vi "Set_CC_Get_Voltage.vi"(7 "Stop Maker 2":dbl=3.0 format="%#_13g", 8 "error in (no error)":errorcluster, 9 "Limit (1.0 A)":dbl=-0.2 format="%.10f", 10 "Channel Name (1)":string, 11 "VISA Refnum in":refnum<visa-resource-name>) -> (0 "error out":errorcluster {"code" format="%.0x"}, 1 "Current Measurement":dbl format="%.10f", 2 "Voltage Measurement":dbl format="%.3f", 3 "VISA Refnum out":refnum<visa-resource-name>)   [LabVIEW 2015]
uses:
  <instrlib>/Agilent N6700 Series/Agilent N6700 Series.lvlib
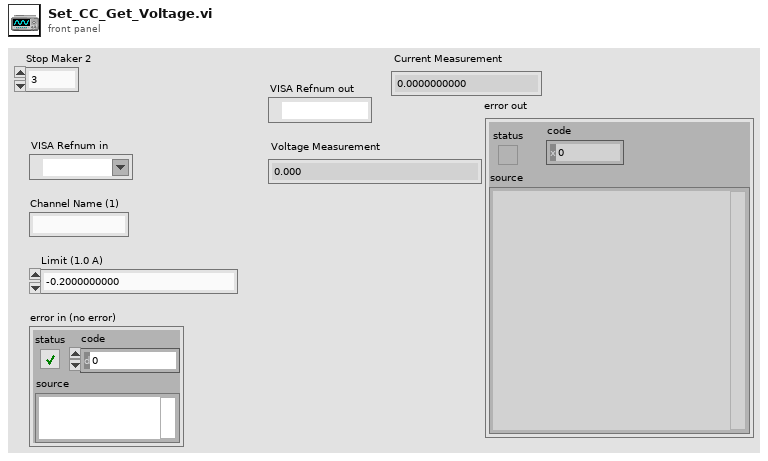
[diagram p1: front panel]
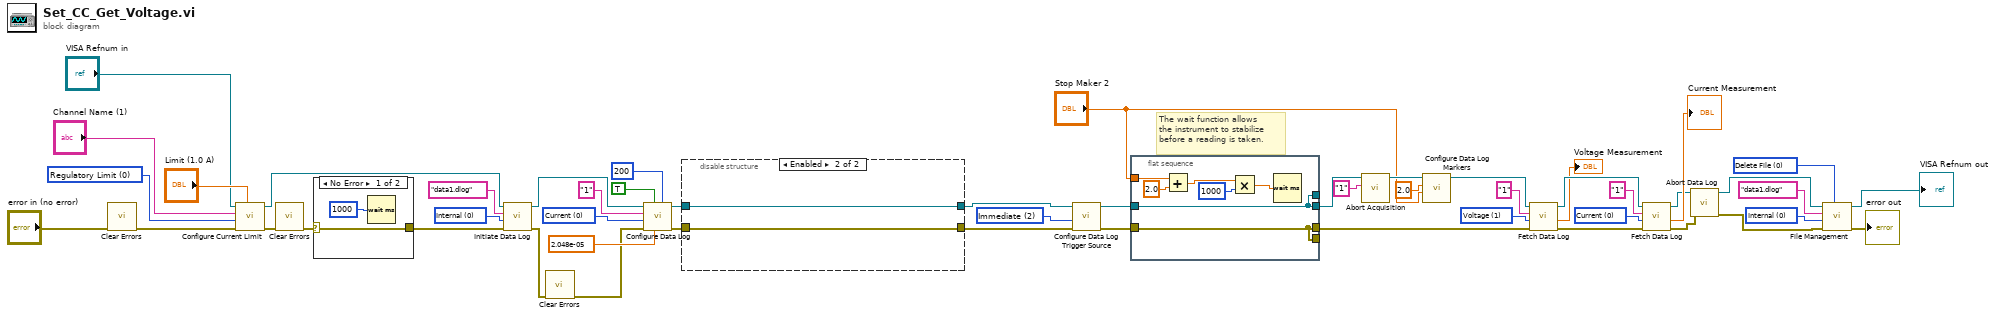
[diagram p0: block diagram]
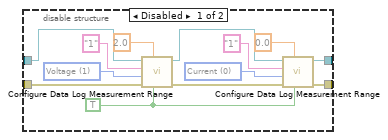
[diagram p3: hidden frame]
diagram:
  w12 = 0 items=["Delete File", "Export Data Log"] ("Operation (1: Export Data Log)")
  w13 = 0 items=["Internal", "External"] ("File Location (0: Internal)")
  w26 = 0 items=["Voltage"=1, "Current"=0] ("Data Log Type (1: Voltage)")
  w34 = 1 items=["Voltage"=1, "Current"=0] ("Data Log Type (1: Voltage)")
  w44 = 2 items=["External", "Software", "Immediate", "Voltage1", "Voltage2", "Voltage3", "Voltage4", "Current1", "Current2", "Current3", "Current4"] ("Data Log Trigger Source (2: Immediate)")
  w41 = 0 items=["Voltage"=1, "Current"=0] ("Data Log Type (1: Voltage)")
  w47 = 0 items=["Internal", "External"] ("Location (0: Internal)")
  w50 = 0 items=["Regulatory Limit", "Trip Limit"] ("Behavior (0: Regulatory Limit)")
  # "The wait function allows \nthe instrument to stabilize\nbefore a reading is taken."
  n1 = call <vilib>:"Clear Errors.vi"("error in (no error)"="error in (no error)") -> ("error out"=w2:errorcluster)  [unwired: 5 in, 1 out]
  n2 = call <instrlib>:"Configure Current Limit.vi"("Limit (0.0 amps)"="Limit (1.0 A)", "error in (no error)"=w2, "Behavior (0: Regulatory Limit)"=w50, "Channel Name (1)"="Channel Name (1)", "VISA resource name"="VISA Refnum in") -> ("error out"=w51:errorcluster, "VISA resource name out"=w20:refnum<visa-resource-name>)  [unwired: 5 in]
  n3 = call <vilib>:"Clear Errors.vi"("error in (no error)"=w51) -> ("error out"=w17:errorcluster)  [unwired: 5 in, 1 out]
  n4 = case shown="No Error" w17 {
    selector: w17 -> [w53 w54]
    tunnel: [w53 w54] -> w16
    frame No Error {
      n5 = Wait (ms)(milliseconds to wait=u32 1000) -> ()  [unwired: 1 out]
    }
    frame Error {
    }
  }
  n6 = call <instrlib>:"Initiate Data Log.vi"("error in (no error)"=w16, "Location (0: Internal)"=w47, "Data Log File Path (data1.dlog)"="data1.dlog", "VISA resource name"=w20) -> ("error out"=w4:errorcluster, "VISA resource name out"=w19:refnum<visa-resource-name>)  [unwired: 6 in]
  n7 = call <vilib>:"Clear Errors.vi"("error in (no error)"=w4) -> ("error out"=w3:errorcluster)  [unwired: 5 in, 1 out]
  n8 = call <instrlib>:"Configure Data Log.vi"("Data Log Duration (30 s)"=200, "Data Log Period (0.1 s)"=2.048e-05, "Enable Data Log (True)"=TRUE, "error in (no error)"=w3, "Data Log Type (1: Voltage)"=w41, "Channel Name (1)"="1", "VISA resource name"=w19) -> ("error out"=w37:errorcluster, "VISA resource name out"=w38:refnum<visa-resource-name>)  [unwired: 3 in]
  n9 = disable-structure shown="Enabled" {
    disable-tunnel: [w67 w69] -> w46
    disable-tunnel: [w66 w68] -> w45
    disable-tunnel: w38 -> [w57 w69]
    disable-tunnel: w37 -> [w56 w68]
    frame Disabled {
      w59 = 0 items=["Voltage"=1, "Current"=0] ("Data Log Type (1: Voltage)")
      w60 = TRUE ("Data Log Auto Range (False)")
      w64 = 1 items=["Voltage"=1, "Current"=0] ("Data Log Type (1: Voltage)")
      n10 = call <instrlib>:"Configure Data Log Measurement Range.vi"("Data Log Auto Range (False)"=w60, "Data Log Measurement Range (0.0)"=2.0, "error in (no error)"=w56, "Data Log Type (1: Voltage)"=w64, "Channel Name (1)"="1", "VISA resource name"=w57) -> ("error out"=w58:errorcluster, "VISA resource name out"=w62:refnum<visa-resource-name>)  [unwired: 4 in]
      n11 = call <instrlib>:"Configure Data Log Measurement Range.vi"("Data Log Auto Range (False)"=w60, "Data Log Measurement Range (0.0)"=0.0, "error in (no error)"=w58, "Data Log Type (1: Voltage)"=w59, "Channel Name (1)"="1", "VISA resource name"=w62) -> ("error out"=w66:errorcluster, "VISA resource name out"=w67:refnum<visa-resource-name>)  [unwired: 4 in]
    }
    frame Enabled {
    }
  }
  n12 = call <instrlib>:"Configure Data Log Trigger Source.vi"("error in (no error)"=w45, "Data Log Trigger Source (2: Immediate)"=w44, "VISA resource name"=w46) -> ("error out"=w30:errorcluster, "VISA resource name out"=w31:refnum<visa-resource-name>)  [unwired: 7 in]
  n13 = flat-sequence {
    tunnel: [w76] -> _
    tunnel: [w76] -> w33
    tunnel: [w75] -> w35
    tunnel: [w75] -> _
    tunnel: w31 -> [w76]
    tunnel: w30 -> [w75]
    tunnel: "Stop Maker 2" -> [w72]
    frame #0 {
      n14 = Add(x=w72, y=2.0) -> (x+y=w70:dbl)
      n15 = Multiply(x=w70, y=u32 1000) -> (x*y=w74:dbl)
      n16 = Wait (ms)(milliseconds to wait=w74) -> ()  [unwired: 1 out]
    }
  }
  n17 = call <instrlib>:"Abort Acquisition.vi"("Channel Name (1)"="1", "VISA resource name"=w33) -> ("VISA resource name out"=w28:refnum<visa-resource-name>)  [unwired: 8 in, 1 out]
  n18 = call <instrlib>:"Configure Data Log Markers.vi"("Data Log Marker 2 (27.5 s)"="Stop Maker 2", "Data Log Marker 1 (7.5 s)"=2.0, "VISA resource name"=w28) -> ("VISA resource name out"=w27:refnum<visa-resource-name>)  [unwired: 7 in, 1 out]
  n19 = call <instrlib>:"Fetch Data Log.vi"("error in (no error)"=w35, "Data Log Type (1: Voltage)"=w34, "Channel Name (1)"="1", "VISA resource name"=w27) -> ("error out"=w23:errorcluster, "Peak to Peak"=→"Voltage Measurement":dbl, "VISA resource name out"=w25:refnum<visa-resource-name>)  [unwired: 5 in]
  n20 = call <instrlib>:"Fetch Data Log.vi"("error in (no error)"=w23, "Data Log Type (1: Voltage)"=w26, "Channel Name (1)"="1", "VISA resource name"=w25) -> ("error out"=w6:errorcluster, "Peak to Peak"=→"Current Measurement":dbl, "VISA resource name out"=w9:refnum<visa-resource-name>)  [unwired: 5 in]
  n21 = call <instrlib>:"Abort Data Log.vi"("error in (no error)"=w6, "VISA resource name"=w9) -> ("error out"=w7:errorcluster, "VISA resource name out"=w8:refnum<visa-resource-name>)  [unwired: 8 in]
  n22 = call <instrlib>:"File Management.vi"("Operation (1: Export Data Log)"=w12, "error in (no error)"=w7, "File Location (0: Internal)"=w13, "File Path"="data1.dlog" ("Data Log File Path (data1.dlog)"), "VISA resource name"=w8) -> ("error out"=→"error out":errorcluster, "VISA resource name out"=→"VISA Refnum out":refnum<visa-resource-name>)  [unwired: 5 in]
